vi "Log Data.vi"(0 "Logging Configuration":T1, 5 "Queue A - Processing":refnum<queue>, 7 "Queue C - DB Results":refnum<queue>, 11 "error in (no error)":errorcluster) -> (15 "error out":errorcluster)   [LabVIEW 2026, in "Processing_Engine.lvlib"]
doc: "This VI uses the TDMS Write function to write data to a TDMS file."
uses:
  Processing_Engine.lvlib
  Processing Configuration.ctl
  controls/Messaging Payloads/Processed Calibration Point.ctl
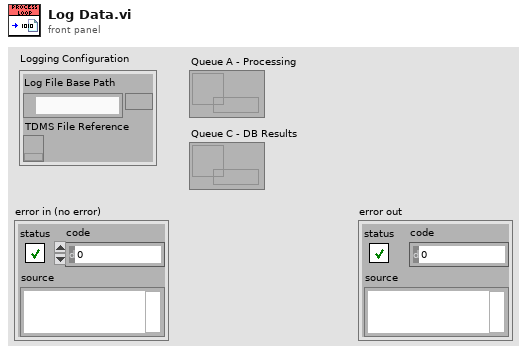
[diagram p1: front panel]
types:
  T1 = typedef "Processing_Engine.lvlib/Processing Configuration.ctl" = cluster{"Log File Base Path":path, "TDMS File Reference":refnum<k34>}
  T2 = typedef "Processed Calibration Point.ctl" = cluster{"Setpoint":dbl, "Measured Value":dbl, "Error":dbl, "Pass/Fail":bool}
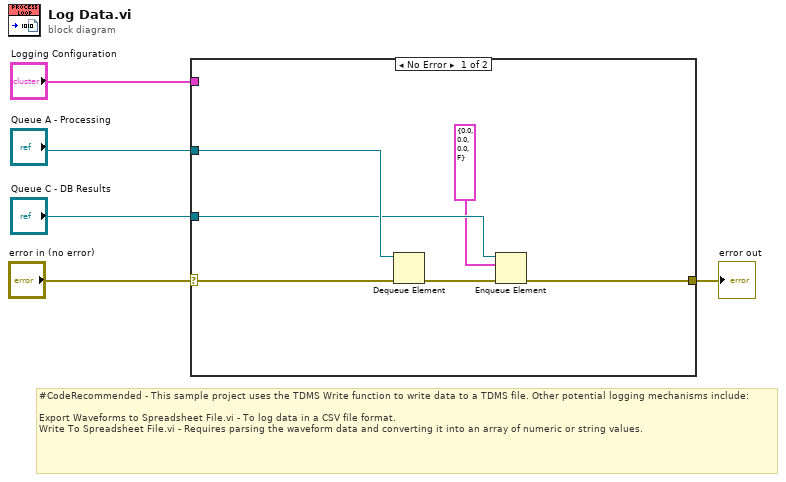
[diagram p0: block diagram]
diagram:
  # "#CodeRecommended - This sample project uses the TDMS Write function to write data to a TDMS file. Other potential logging mechanisms include:\n\nExport Waveforms to Spreadsheet File.vi - To log data in a CSV file format.\nWrite To Spreadsheet File.vi - Requires parsing the waveform data and converting it into an array of numeric or string values."
  n1 = case shown="No Error" "error in (no error)" {
    selector: "error in (no error)" -> [w11 w12]
    tunnel: "Logging Configuration" -> [_ _]
    tunnel: "Queue C - DB Results" -> [w7 _]
    tunnel: [w8 w12] -> w4
    tunnel: "Queue A - Processing" -> [w10 _]
    frame No Error {
      n2 = Dequeue Element(queue=w10, error in (no error)=w11) -> (error out=w9:errorcluster)  [unwired: 1 in, 3 out]
      n3 = Enqueue Element(queue=w7, element=T2 {"Setpoint"=0.0, "Measured Value"=0.0, "Error"=0.0, "Pass/Fail"=FALSE}, error in (no error)=w9) -> (error out=w8:errorcluster)  [unwired: 1 in, 2 out]
    }
    frame Error {
    }
  }
  "error out" <- w4
